vi "Render Text-Comment.vi"(8 "Error In":errorcluster) -> (0 "Error Out":errorcluster)   [LabVIEW 2018, in "Tests.lvlib" / "Render.lvlib"]
uses:
  Render.lvlib
  src/Toolkit/Data/Null/Null.lvclass
  D:/Users/cfield/Code/Field R&D Services/Mustache/trunk/src/Toolkit/Data/Abstract/Abstract.lvclass
  src/Toolkit/Low-Level/Support/Lex String.vi
  src/Toolkit/Low-Level/Support/Render to String.vi
  <vilib>/addons/_JKI Toolkits/Caraya/classes/Test/Test.lvclass
  <vilib>/addons/_JKI Toolkits/Caraya/classes/Assert/Assert.lvclass
  src/Toolkit/Toolkit.lvlib
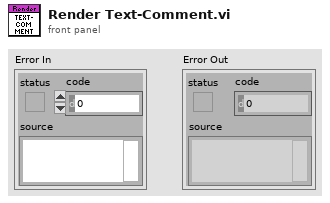
[diagram p1: front panel]
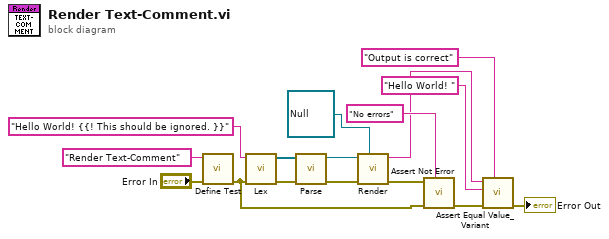
[diagram p0: block diagram]
diagram:
  n1 = call <vilib>:"Define Test.vi"("error in (no error)"="Error In", "Label (VI Title)"="Render Text-Comment") -> ("error out"=w5:errorcluster)  [unwired: 9 in]
  n2 = call-poly "Lex.vi"("Error In"=w5, "Input"="Hello World! {{! This should be ignored. }}") -> ("Error Out"=w6:errorcluster, "Tokens"=w7:refnum<class "Abstract.lvclass">[])  [unwired: 8 in]
  n3 = call "Parse.vi"("Error In"=w6, "Tokens"=w7) -> ("Error Out"=w8:errorcluster, "Abstract Syntax Tree"=w4:refnum<class "Root.lvclass">)  [unwired: 8 in]
  n4 = call-poly "Render.vi"("Data"=refnum<class "Null.lvclass"> refnum ("Toolkit.lvlib:Data.lvlib:Null.lvclass"), "Error In"=w8, "Abstract Syntax Tree"=w4) -> ("Error Out"=w10:errorcluster, "Output"=w9:string)  [unwired: 7 in]
  n5 = call <vilib>:"Assert Not Error.vi"("Label"="No errors", "error in (no error)"=w5, "Not Error?"=w10) -> ("error out"=w13:errorcluster)  [unwired: 8 in]
  n6 = call <vilib>:"Assert Equal Value_Variant.vi"("Label"="Output is correct", "error in (no error)"=w13, "Y"="Hello World! ", "X"=w9) -> ("error out"=→"Error Out":errorcluster)  [unwired: 7 in]
